vi "onAssertionSlippage.vi"(7 "AssertEqualType in":refnum<class "AssertEqualType.lvclass">, 11 "Leaf.Assertion":refnum<class "Leaf.Assertion.lvclass">) -> (0 "error out":errorcluster, 3 "Leaf.Assertion":refnum<class "Leaf.Assertion.lvclass">)   [LabVIEW 2021, in "Bananas.lvlib" / "AssertEqualType.lvclass"]
uses:
  AssertEqualType.lvclass
  <vilib>/addons/_JKI Toolkits/Caraya/classes/Properties.Assert/Properties.Assert.lvclass/Properties.Assert.ctl
  AssertEqualType.lvclass/AssertEqualType.ctl
  Read Not_.vi
  Read Y.vi
  Read X.vi
  Bananas.lvlib
  <vilib>/Utility/Data Type/NI_Data Type.lvlib
  Leaf.Assertion/Leaf.Assertion.lvclass
  Leaf/Leaf.lvclass
  C:/Repositories/LVOS/Bananas/lv-src/Bananas/Leaf.Assertion/Leaf.Assertion.lvclass
  C:/Repositories/LVOS/Bananas/lv-src/Bananas/Leaf/Leaf.lvclass
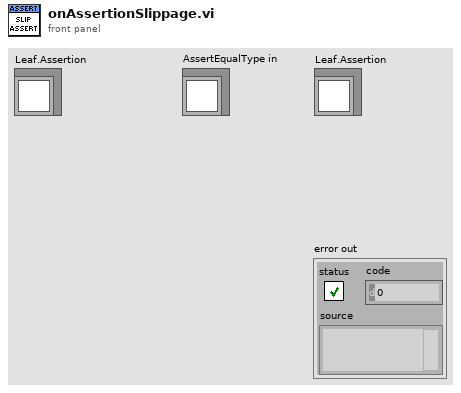
[diagram p1: front panel]
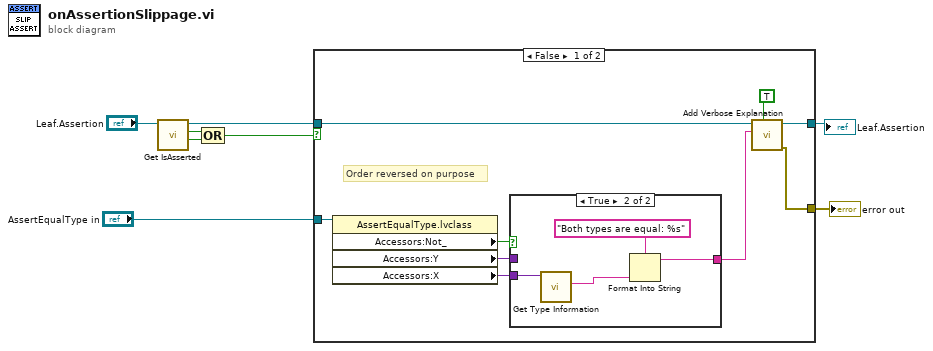
[diagram p0: block diagram]
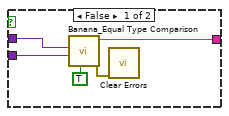
[diagram p2: hidden frame]
diagram:
  n1 = call "Get IsAsserted.vi"("Leaf.Assertion"="Leaf.Assertion") -> ("UpstreamError"=w4:bool, "Asserted"=w5:bool, "Leaf.Assertion"=w2:refnum<class "Leaf.Assertion.lvclass">)  [unwired: 8 in]
  n2 = Compound Arithmetic op=OR(w5, w4) -> (w1:bool)
  n3 = case shown="False" w1 {
    tunnel: [w11 w27] -> w8
    tunnel: [w10 _] -> w7
    tunnel: w2 -> [w13 w27]
    tunnel: "AssertEqualType in" -> [w17 _]
    frame False {
      # "Order reversed on purpose"
      n4 = property class="AssertEqualType.lvclass"(reference=w17) -> ("Accessors:Not_"=w14:bool, "Accessors:Y"=w16:variant, "Accessors:X"=w15:variant)  [unwired: 1 in, 2 out]
      n5 = case shown="True" w14 {
        tunnel: w16 -> [w22 _]
        tunnel: w15 -> [w21 w26]
        tunnel: [w20 w24] -> w9
        frame False {
          n6 = call "Banana_Equal Type Comparison.vi"("verbose? (F)"=TRUE, "Y"=w21, "X"=w22) -> ("error out"=w19:errorcluster, "Verbose output"=w20:string)  [unwired: 6 in, 1 out]
          n7 = call <vilib>:"Clear Errors.vi"("error in (no error)"=w19) -> ()  [unwired: 5 in, 2 out]
        }
        frame True {
          n8 = call <vilib>:"Get Type Information.vi"("variant"=w26) -> ("name"=w23:string)  [unwired: 6 in, 4 out]
          n9 = Format Into String(format string="Both types are equal: %s" ("Verbose output"), w23) -> (resulting string=w24:string)  [unwired: 2 in, 1 out]
        }
      }
      n10 = call "Add Verbose Explanation.vi"("overwrite"=TRUE ("overwrite?"), "Verbose Explanation"=w9, "Leaf in"=w13) -> ("error out"=w10:errorcluster, "Leaf out"=w11:refnum<class "Leaf.Assertion.lvclass">)  [unwired: 7 in]
    }
    frame True {
      # "There was an upstream error or the assertion = TRUE"
    }
  }
  "error out" <- w7
  "Leaf.Assertion" <- w8
